vi "Lookup_Table_Map_Shooter.vi"(1 "x":dbl, 2 "X_Array":dbl[](array[numeric]), 3 "Y-Array":dbl[](array[numeric])) -> (0 "Y":dbl)   [LabVIEW 2019]
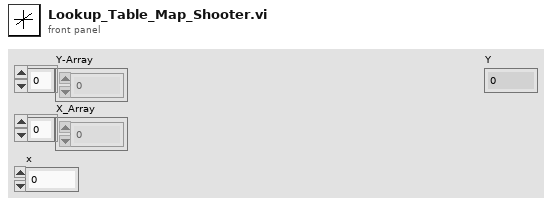
[diagram p1: front panel]
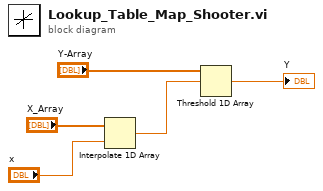
[diagram p0: block diagram]
diagram:
  n1 = Interpolate 1D Array(1:"x", 2:"X_Array") -> (0:w5:dbl)
  n2 = Threshold 1D Array(2:w5, 3:"Y-Array") -> (0:→"Y":dbl)  [unwired: 1 in]
